vi "Find setpoint.vi"(0 "reference in":refnum<class "Force Curve_tdms.lvclass">, 5 "error in (no error)":errorcluster, 7 "Signal in":T1=enum."SensorIn") -> (14 "reference out":refnum<class "Force Curve_tdms.lvclass">, 16 "Setpoint index":i32, 19 "error out":errorcluster)   [LabVIEW 2019, in "Force Curve_tdms.lvclass"]
uses:
  Force Curve_tdms.lvclass
  Signal In.ctl
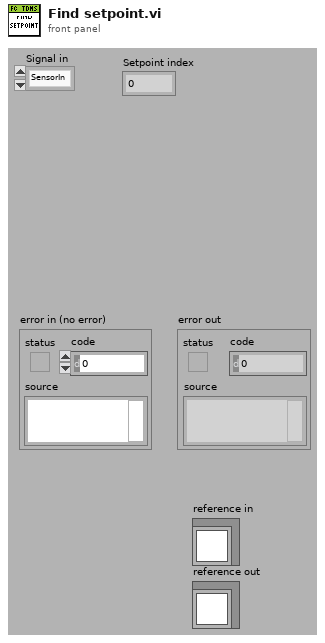
[diagram p1: front panel]
types:
  T1 = typedef "Force Curve_tdms.lvclass/Signal In.ctl" = enum16{"Deflection", "SensorIn", "MockOut", "ZstageOut"}
  T2 = typedef "Force Curve_tdms.lvclass/ObjectAttributes.ctl" = cluster{"MyAttribute":dbl, "Processed data":waveform(dbl)[], "Fcurve Raw Metadata":T3, "Fcurve Metadata":T4, "Fcurve index":T5, "Tau Delay (ms)":dbl, "Contact Spread of dev":dbl, "Fcurve":T6}
  T3 = typedef "TDMS_DataHandler.lvclass/Fcurve Meta data.ctl" = cluster{"property names":string[], "property values":variant[]}
  T4 = typedef "Force Curve_tdms.lvclass/Fcurve Meta data analysis.ctl" = cluster{"dt (us)":dbl, "Dec Factor":dbl, "Z piezo Sensitivity (nm/V)":dbl, "K (N/m)":dbl, "Sp (V)":dbl, "Contact (ms)":dbl, "Zpos contact":dbl, "Vel_app (nm/s)":dbl, "Vel_ret (nm/s)":dbl, "deltaV (nm)":dbl, "Def_V0 (v)":dbl, "Decimating Factor":dbl}
  T5 = typedef "Force Curve_tdms.lvclass/Fcurve Index .ctl" = cluster{"Setpoint index":i32, "Max force index":i32, "Contact point index":i32, "Appoach indices":cluster{"Start":i32, "End":i32}, "Contact indices":cluster{"Start":i32, "End":i32}, "Retract indices":cluster{"Start":i32, "End":i32}}
  T6 = typedef "Force Curve_tdms.lvclass/Force Curve data.ctl" = cluster{"Approach":cluster{"X":dbl[], "Y":dbl[]}, "Contact":cluster{"X":dbl[], "Y":dbl[]}, "Retract":cluster{"X":dbl[], "Y":dbl[]}}
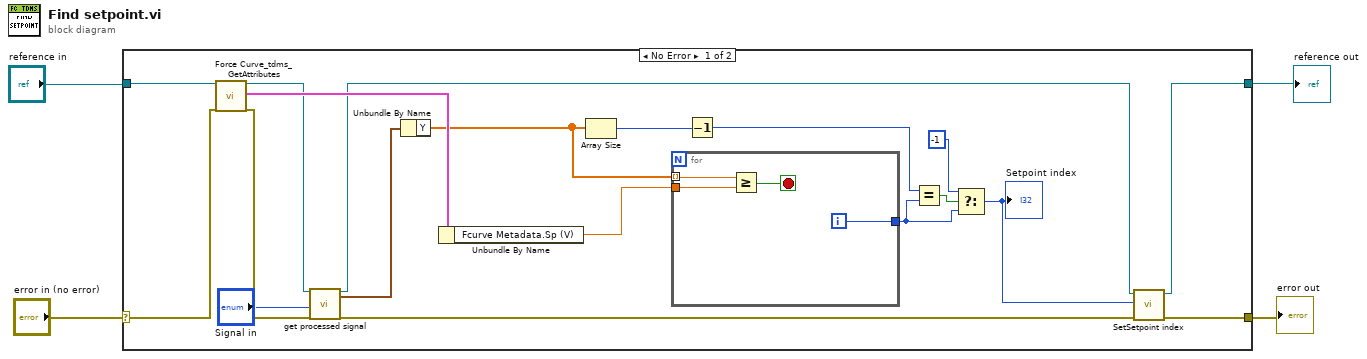
[diagram p0: block diagram]
diagram:
  n1 = case shown="No Error" "error in (no error)" {
    selector: "error in (no error)" -> [w18 w29]
    tunnel: [w8 w29] -> w3
    tunnel: "reference in" -> [w17 w28]
    tunnel: [w6 w28] -> w1
    frame No Error {
      n2 = call "Force Curve_tdms_GetAttributes.vi"("reference in"=w17, "error in (no error)"=w18) -> ("reference out"=w10:refnum<class "Force Curve_tdms.lvclass">, "attributes"=w16:T2, "error out"=w14:errorcluster)  [unwired: 14 in, 1 out]
      n3 = call "get processed signal.vi"("reference in"=w10, "error in (no error)"=w14, "Signal in"="Signal in") -> ("reference out"=w7:refnum<class "Force Curve_tdms.lvclass">, "Wfm out"=w11:waveform(dbl), "error out"=w9:errorcluster)  [unwired: 14 in]
      n4 = Unbundle By Name(w11) -> ("Y"=w13:dbl[])
      n5 = Unbundle By Name(w16) -> ("Fcurve Metadata.Sp (V)"=w15:dbl)
      n6 = Array Size(array=w13) -> (size(s)=w23:i32)
      n7 = for {
        tunnel: w13 -> [w27] mode=indexing
        tunnel: w15 -> [w26]
        tunnel: [w24] -> w20
        i -> [w24]
        stop <- w25 stop-if-true
        n8 = Greater Or Equal?(x=w27, y=w26) -> (x >= y?=w25:bool)
      }
      n9 = Decrement(x=w23) -> (x-1=w22:i32)
      n10 = Equal?(x=w22, y=w20) -> (x = y?=w21:bool)
      n11 = Select(t=-1, s=w21, f=w20) -> (s? t:f=w5:i32)
      "Setpoint index" <- w5
      n12 = call-dynamic "SetSetpoint index.vi"("error in (no error)"=w9, "Setpoint index"=w5, "reference in"=w7) -> ("error out"=w8:errorcluster, "reference out"=w6:refnum<class "Force Curve_tdms.lvclass">)  [unwired: 7 in]
    }
    frame Error {
    }
  }
  "error out" <- w3
  "reference out" <- w1
